vi "Set Extension.vi"(8 "error in (no error)":errorcluster, 11 "TXT_Report":refnum<class "Wind TXT Report.lvclass">) -> (0 "error out":errorcluster, 3 "TXT_Report out":refnum<class "Wind TXT Report.lvclass">)   [LabVIEW 2009, in "Wind TXT Report.lvclass"]
doc: "This dynamic dispatch VI overrides the parent and sets the unique file extension for the child class.\n\nAAL 9/09"
uses:
  Wind TXT Report.lvclass
  Wind Report/Wind Report.lvclass
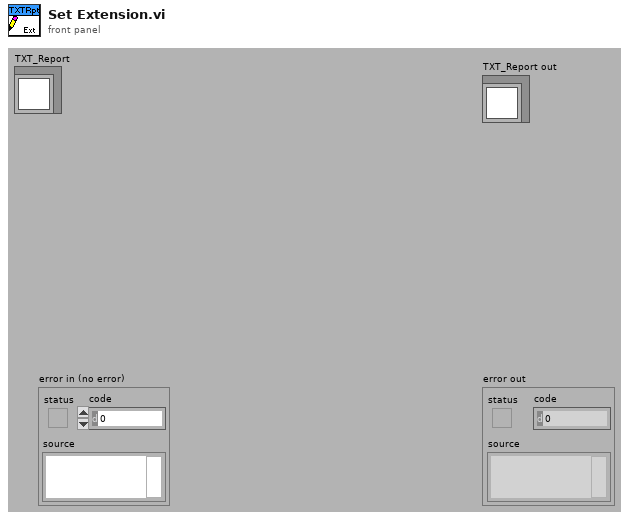
[diagram p1: front panel]
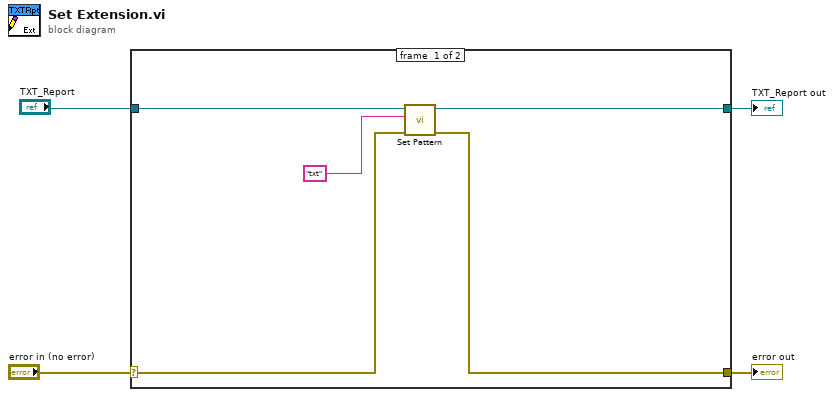
[diagram p0: block diagram]
diagram:
  n1 = case shown="No Error" "error in (no error)" {
    selector: "error in (no error)" -> [w7 w11]
    tunnel: [w6 w11] -> w3
    tunnel: [w9 w10] -> w2
    tunnel: "TXT_Report" -> [w5 w10]
    frame #0 {
      n2 = call "Set Pattern.vi"("error in (no error)"=w7, "Pattern"="txt", "Report.lvclass in"=w5) -> ("error out"=w6:errorcluster, "Report.lvclass out"=w9:refnum<class "Wind TXT Report.lvclass">)  [unwired: 7 in]
    }
    frame #1 {
    }
  }
  "error out" <- w3
  "TXT_Report out" <- w2
